vi "build_en_face_interp_sequential.vi"(0 "Existing En Face":T1, 1 "Image to add":T1, 2 "current x":i32, 3 "current y":i32, 4 "depth":i32, 5 "error in (no error)":errorcluster, 6 "add height":dbl, 7 "output line":dbl, 9 "Track Surface":bool) -> (14 "En Face Image Out":T1)   [LabVIEW 2016]
doc: "Adds line or group of lines to image."
uses:
  <vilib>/vision/Image Controls.llb/IMAQ Image.ctl
panel:
  out "error out":errorcluster
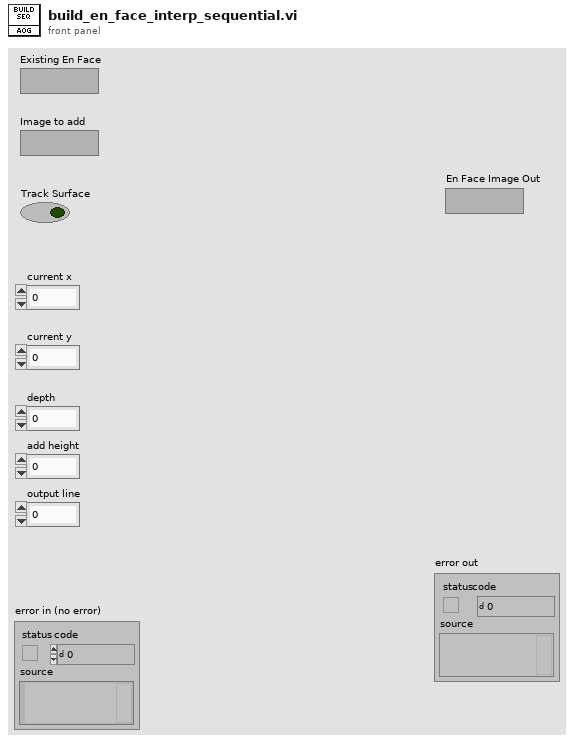
[diagram p1: front panel]
types:
  T1 = typedef "IMAQ Image.ctl" = refnum<image>
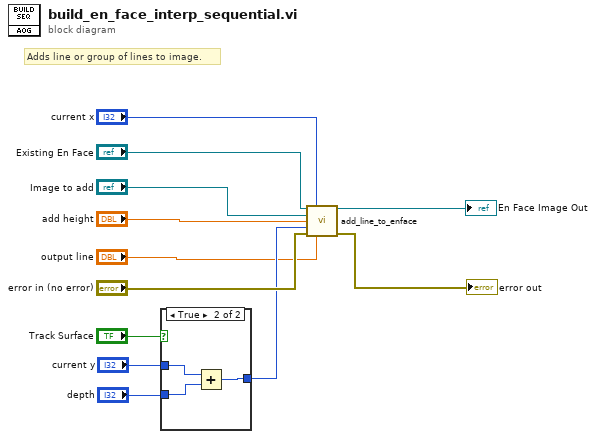
[diagram p0: block diagram]
diagram:
  # "Adds line or group of lines to image."
  n1 = case shown="True" "Track Surface" {
    tunnel: "depth" -> [w13 w16]
    tunnel: "current y" -> [_ w15]
    tunnel: [w13 w14] -> w3
    frame False {
    }
    frame True {
      n2 = Add(x=w15, y=w16) -> (x+y=w14:i32)
    }
  }
  n3 = call "add_line_to_enface.vi"("En Face Image"="Existing En Face", "Shift"="current x", "Raw Image"="Image to add", "Add Height"="add height", "Input Line"=w3, "error in (no error)"="error in (no error)", "Output Line"="output line") -> ("En Face Image Out"=→"En Face Image Out":T1, "error out"=→"error out":errorcluster)  [unwired: 7 in]
